vi "instrument.vi"(4 "center":cluster{"x":i32, "y":i32}={"x"=35, "y"=32}, 5 "stabile":bool=TRUE, 6 "size":i16=29, 7 "plane control":T1={"control stick"={"roll"=0, "pitch"=0}, "rotate"={"pitch"=1.3766765505351941e-14, "roll"=2.6645352591003757e-15, "yaw"=2.6645352591003757e-15}, "pos"={"x"=1.1102230246251565e-15, "y"=0.0, "z"=0}} {"rotate"."pitch" scale=-180.0..180.0; "rotate"."roll" scale=-180.0..180.0; "rotate"."yaw" scale=-180.0..180.0; "pos"."x" scale=0.0..10.0; "pos"."y" scale=0.0..100.0; "pos"."z" scale=0.0..10.0}) -> (2 "pict out":picture)   [LabVIEW 2017]
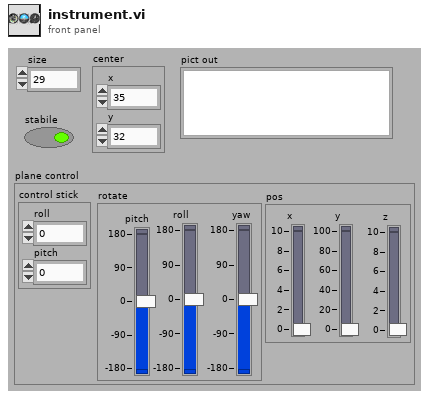
[diagram p1: front panel]
types:
  T1 = cluster{"control stick":cluster{"roll":i32, "pitch":i32}, "rotate":cluster{"pitch":dbl, "roll":dbl, "yaw":dbl}, "pos":cluster{"x":dbl, "y":dbl, "z":i32}}
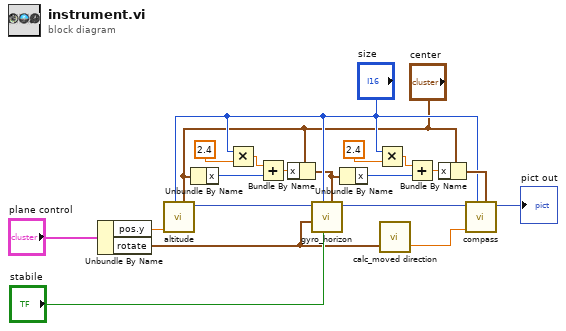
[diagram p0: block diagram]
diagram:
  n1 = Unbundle By Name("plane control") -> ("pos.y"=w1:dbl, "rotate"=w2:cluster{"pitch":dbl, "roll":dbl, "yaw":dbl})
  n2 = call "altitude.vi"("center"="center", "size"="size", "altitude"=w1) -> ("pict out"=w12:picture)  [unwired: 7 in]
  n3 = Unbundle By Name("center") -> ("x"=w10:i32)
  n4 = Multiply(x="size", y=2.4) -> (x*y=w9:dbl)
  n5 = Add(x=w9, y=w10) -> (x+y=w11:dbl)
  n6 = Bundle By Name(cluster="center", "x"=w11) -> (w6:cluster{"x":i32, "y":i32})
  n7 = call "gyro_horizon.vi"("center"=w6, "stabile"="stabile", "size"="size", "rotate"=w2, "pict in"=w12) -> ("gyro_horizon"=w14:picture)  [unwired: 6 in]
  n8 = Unbundle By Name(w6) -> ("x"=w18:i32)
  n9 = Multiply(x="size", y=2.4) -> (x*y=w19:dbl)
  n10 = call "calc_moved direction.vi"("rotate"=w2) -> ("compass angle"=w4:dbl)  [unwired: 1 in, 1 out]
  n11 = Add(x=w19, y=w18) -> (x+y=w17:dbl)
  n12 = Bundle By Name(cluster="center", "x"=w17) -> (w16:cluster{"x":i32, "y":i32})
  n13 = call "compass.vi"("center"=w16, "size"="size", "angle"=w4, "pict in"=w14) -> ("pict out"=→"pict out":picture)  [unwired: 6 in]
